vi "NIDMM_Initialize.vi"(8 "error in (no error)":errorcluster, 10 "Reset":bool=TRUE, 11 "Instrument Descriptor":refnum<k15>="NI_DMM") -> (0 "error out":errorcluster)   [LabVIEW 2015]
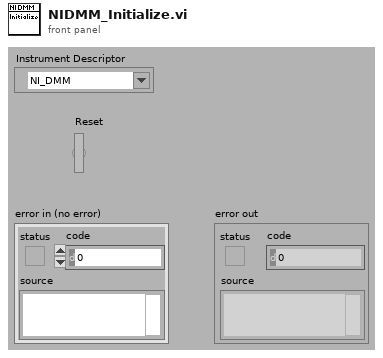
[diagram p1: front panel]
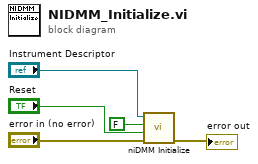
[diagram p0: block diagram]
diagram:
  n1 = call <instrlib>:"niDMM Initialize.vi"("error in (no error)"="error in (no error)", "Reset"="Reset", "ID Query"=FALSE ("id query (True)"), "Instrument Descriptor"="Instrument Descriptor") -> ("error out"=→"error out":errorcluster)  [unwired: 6 in, 1 out]
